vi "EtherNet_IP Update Registers.vi"(3 "error in":errorcluster, 4 "Registers":u16[](array[numeric]), 5 "Offset(N7:?)":u8, 6 "Connection Cluster":T1={"TCP Connection"=refnum, "Session"=[], "EtherNet/IP Device Address"="172.20.37.243"} {"Session" format="0x%02x"}) -> (0 "error out":errorcluster, 1 "Data Error":bool, 2 "Connection Cluster Out":T1)   [LabVIEW 2020, in "EtherNet_IP_Lib.lvlib"]
uses:
  EtherNet_IP_Lib.lvlib
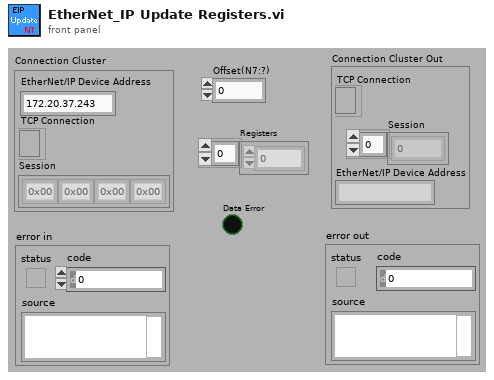
[diagram p1: front panel]
types:
  T1 = cluster{"TCP Connection":refnum<k5>, "Session":u8[], "EtherNet/IP Device Address":string}
  T2 = enum16{"Standard", "Buffered", "CRLF", "Immediate"}
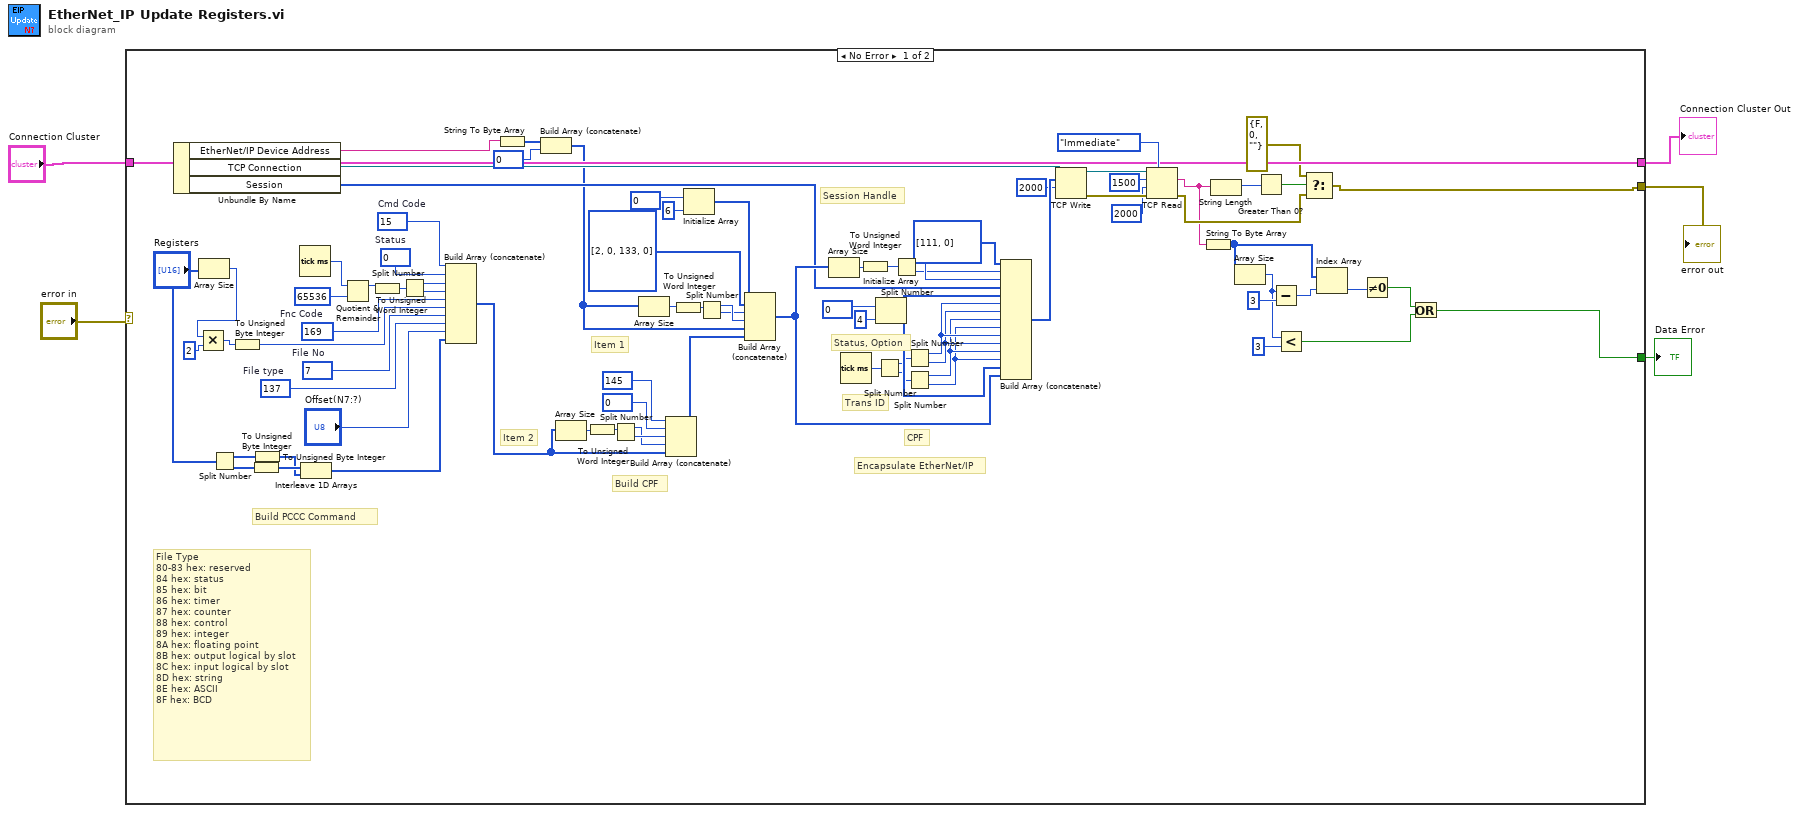
[diagram p0: block diagram]
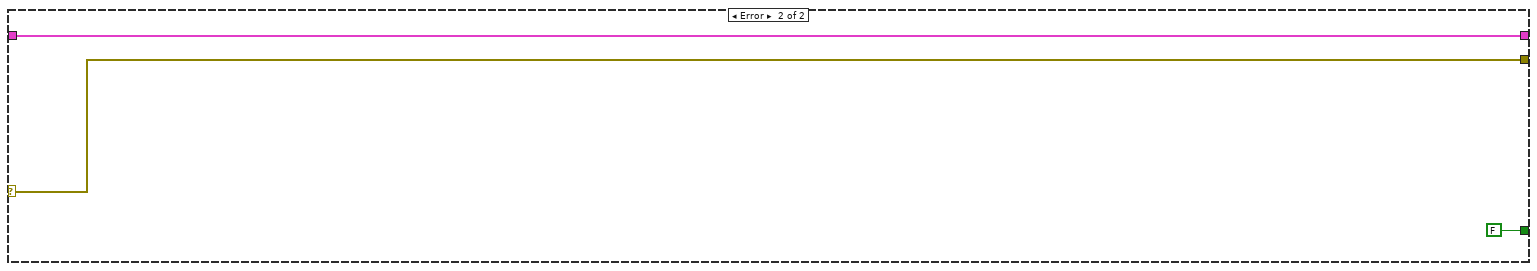
[diagram p2: hidden frame]
diagram:
  n1 = case shown="No Error" "error in" {
    selector: "error in" -> [_ w91]
    tunnel: "Connection Cluster" -> [w46 w90]
    tunnel: [w41 w91] -> w5
    tunnel: [w46 w90] -> w2
    tunnel: [w7 FALSE] -> w1
    frame No Error {
      w32 = u8 137  # File type
      w33 = u8 7  # File No
      w34 = u8 169  # Fnc Code
      w81 = u8 0  # Status
      w80 = u8 15  # Cmd Code
      # "File Type\n80-83 hex: reserved\n84 hex: status\n85 hex: bit\n86 hex: timer\n87 hex: counter\n88 hex: control\n89 hex: integer\n8A hex: floating point\n8B hex: output logical by slot\n8C hex: input logical by slot\n8D hex: string\n8E hex: ASCII\n8F hex: BCD"
      # "Build CPF"
      # "Trans ID"
      # "CPF"
      # "Status, Option"
      # "Session Handle"
      # "Item 2"
      # "Item 1"
      # "Encapsulate EtherNet/IP"
      # "Build PCCC Command"
      n2 = Unbundle By Name(w46) -> ("EtherNet/IP Device Address"=w47:string, "TCP Connection"=w85:refnum<k5>, "Session"=w56:u8[])
      n3 = Array Size(array="Registers") -> (size(s)=w25:i32)
      n4 = Multiply(x=w25, y=u8 2) -> (x*y=w18:i32)
      n5 = Split Number(x="Registers") -> (hi(x)=w23:u8[], lo(x)=w22:u8[])
      n6 = To Unsigned Byte Integer(number=w18) -> (unsigned 8bit integer=w17:u8)
      n7 = To Unsigned Byte Integer(number=w22) -> (unsigned 8bit integer=w21:u8[])
      n8 = To Unsigned Byte Integer(number=w23) -> (unsigned 8bit integer=w20:u8[])
      n9 = Tick Count (ms)() -> (millisecond timer value=w76:u32)
      n10 = Interleave 1D Arrays(w21, w20) -> (w19:u8[])
      n11 = Quotient & Remainder(x=w76, y=u32 65536) -> (x-y*floor(x/y)=w78:u32)  [unwired: 1 out]
      n12 = To Unsigned Word Integer(number=w78) -> (unsigned 16bit integer=w79:u16)
      n13 = Split Number(x=w79) -> (hi(x)=w82:u8, lo(x)=w83:u8)
      n14 = Build Array (concatenate)(w80, w81, w82, w83, w34, w17, w33, w32, "Offset(N7:?)", w19) -> (w36:u8[])
      n15 = String To Byte Array(string=w47) -> (unsigned byte array=w74:u8[])
      n16 = Build Array (concatenate)(w74, u8 0 ("Status")) -> (w39:u8[])
      n17 = Array Size(array=w36) -> (size(s)=w73:i32)
      n18 = To Unsigned Word Integer(number=w73) -> (unsigned 16bit integer=w72:u16)
      n19 = Split Number(x=w72) -> (hi(x)=w70:u8, lo(x)=w71:u8)
      n20 = Array Size(array=w39) -> (size(s)=w37:i32)
      n21 = Build Array (concatenate)(u8 145 ("Status"), u8 0 ("Status"), w71, w70, w36) -> (w35:u8[])
      n22 = To Unsigned Word Integer(number=w37) -> (unsigned 16bit integer=w38:u16)
      n23 = Initialize Array(u8 0 ("Status"), 6 ("dimension size")) -> (w65:u8[])
      n24 = Split Number(x=w38) -> (hi(x)=w28:u8, lo(x)=w27:u8)
      n25 = Build Array (concatenate)(w65, u8[] [2, 0, 133, 0], w27, w28, w39, w35) -> (w57:u8[])
      n26 = Array Size(array=w57) -> (size(s)=w63:i32)
      n27 = Tick Count (ms)() -> (millisecond timer value=w55:u32)
      n28 = To Unsigned Word Integer(number=w63) -> (unsigned 16bit integer=w64:u16)
      n29 = Split Number(x=w55) -> (hi(x)=w54:u16, lo(x)=w53:u16)
      n30 = Initialize Array(u8 0 ("Status"), 4 ("dimension size")) -> (w58:u8[])
      n31 = Split Number(x=w64) -> (hi(x)=w62:u8, lo(x)=w61:u8)
      n32 = Split Number(x=w54) -> (hi(x)=w52:u8, lo(x)=w51:u8)
      n33 = Split Number(x=w53) -> (hi(x)=w50:u8, lo(x)=w49:u8)
      n34 = Build Array (concatenate)(u8[] [111, 0], w61, w62, w56, w58, w52, w51, w50, w49, w52, w51, w50, w49, w58, w57) -> (w16:u8[])
      n35 = TCP Write(connection ID=w85, data in=w16, 9:2000 ("timeout ms (25000)")) -> (connection ID out=w87:refnum<k5>, error out=w88:errorcluster)  [unwired: 1 in, 1 out]
      n36 = TCP Read(connection ID=w87, bytes to read=1500, error in (no error)=w88, 7:T2."Immediate" ("mode (standard)"), 9:2000 ("timeout ms (25000)")) -> (data out=w40:string, error out=w42:errorcluster)  [unwired: 1 out]
      n37 = String To Byte Array(string=w40) -> (unsigned byte array=w14:u8[])
      n38 = String Length(string=w40) -> (length=w45:i32)
      n39 = Array Size(array=w14) -> (size(s)=w11:i32)
      n40 = Greater Than 0?(x=w45) -> (x > 0?=w44:bool)
      n41 = Subtract(x=w11, y=3) -> (x-y=w13:i32)
      n42 = Less?(x=w11, y=3) -> (x < y?=w8:bool)
      n43 = Select(t=errorcluster {"status"=FALSE, "code"=0, "source"=""} ("error IO"), s=w44, f=w42) -> (s? t:f=w41:errorcluster)
      n44 = Index Array(array=w14, index=w13) -> (element=w12:u8)
      n45 = Not Equal To 0?(x=w12) -> (x != 0?=w9:bool)
      n46 = Or(x=w9, y=w8) -> (x .or. y?=w7:bool)
    }
    frame Error {
    }
  }
  "error out" <- w5
  "Connection Cluster Out" <- w2
  "Data Error" <- w1
